vi "PostCopyScripting.vi"(10 "MetaDataObj":refnum<class "MetaDataObj.lvclass">, 11 "User Project":refnum<vi>) -> ()   [LabVIEW 2016, in "MeasurementMetaData.lvclass"]
uses:
  MeasurementMetaData.lvclass
  <resource>/dialog/NewProjectWizard/MetaDataObj/MetaDataObj.lvclass
  C:/Program Files (x86)/National Instruments/LabVIEW 2016/resource/dialog/NewProjectWizard/MetaDataObj/MetaDataObj.lvclass
  <resource>/dialog/NewProjectWizard/MetaDataObj/MetaDataObj.lvclass/MetaDataObj.ctl
  MeasurementMetaData.lvclass/MeasurementMetaData.ctl
  <vilib>/Utility/EditLVProj/Edit LVProj.lvlib
  <resource>/dialog/NewProjectWizard/Project Copying/NI_NPW_Project Copying.lvlib
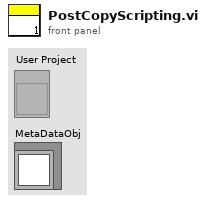
[diagram p1: front panel]
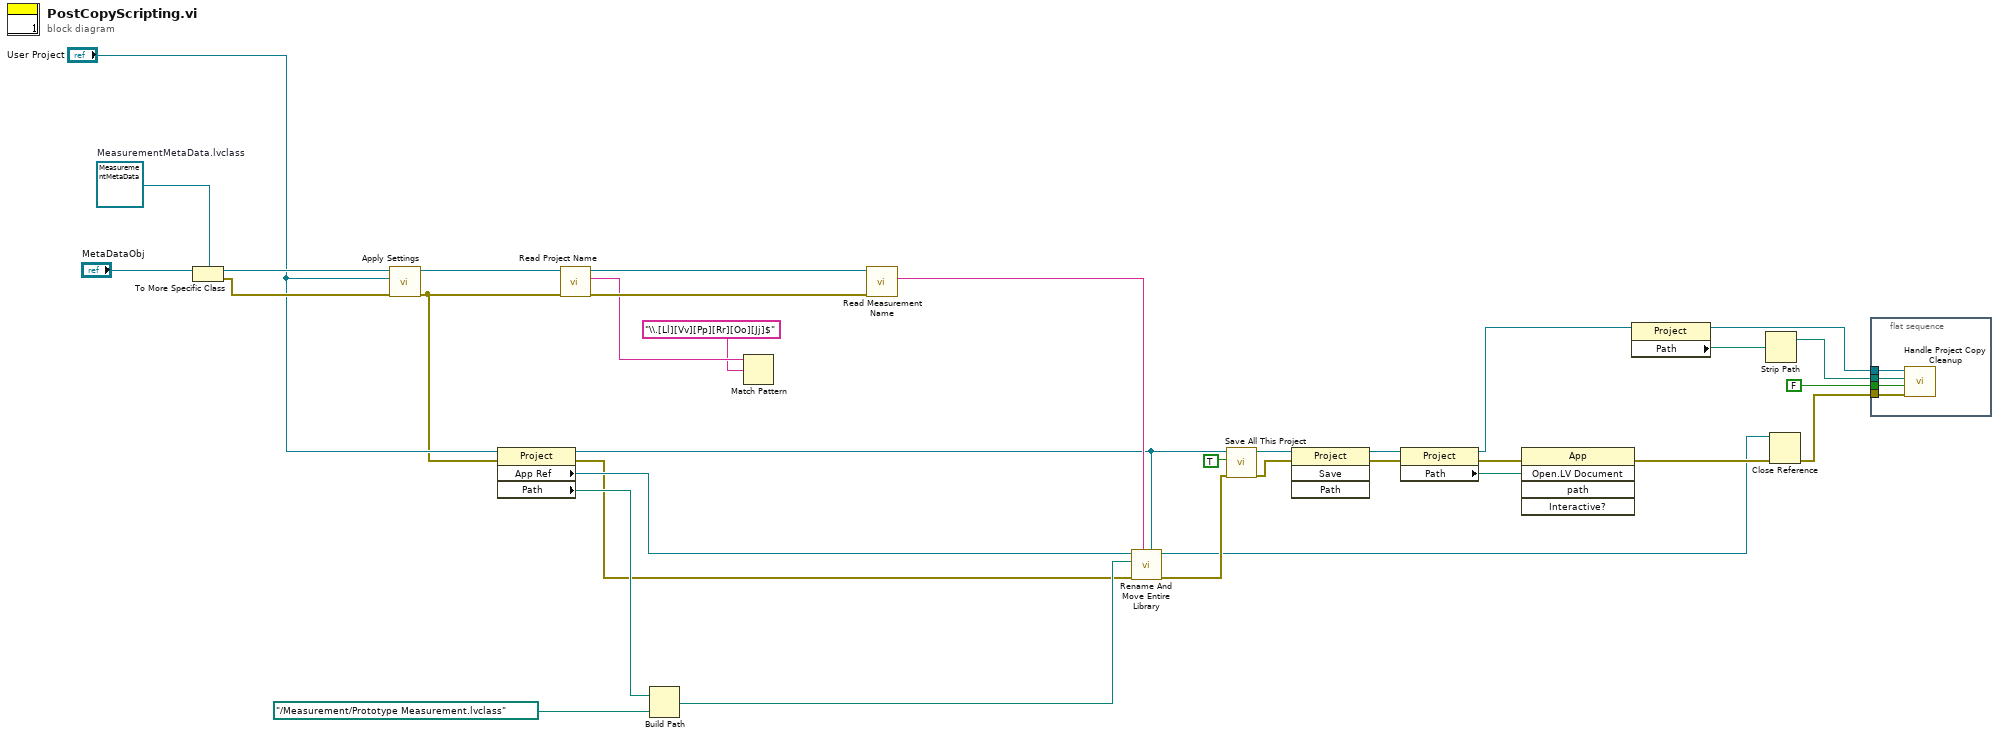
[diagram p0: block diagram]
diagram:
  w34 = refnum<class "MeasurementMetaData.lvclass"> refnum  # MeasurementMetaData.lvclass
  n1 = To More Specific Class(target class=w34, reference="MetaDataObj") -> (specific class reference=w24:refnum<class "MeasurementMetaData.lvclass">, error out=w23:errorcluster)  [unwired: 1 in]
  n2 = call "Apply Settings.vi"("error in (no error)"=w23, "User Project"="User Project", "MeasurementMetaData in"=w24) -> ("error out"=w8:errorcluster, "MeasurementMetaData out"=w10:refnum<class "MeasurementMetaData.lvclass">)  [unwired: 7 in]
  n3 = property class="Project"(reference="User Project", error in=w8) -> (reference out=w6:refnum<vi>, error out=w3:errorcluster, "App Ref"=w5:refnum<vi>, "Path"=w12:path)
  n4 = call <resource>:"Read Project Name.vi"("error in (no error)"=w8, "MetaDataObj in"=w10) -> ("error out"=w19:errorcluster, "Project Name"=w18:string, "MetaDataObj out"=w20:refnum<class "MeasurementMetaData.lvclass">)  [unwired: 7 in]
  n5 = Build Path(base path=w12, name or relative path=path "../Measurement/Prototype Measurement.lvclass" ("Path")) -> (appended path=w4:path)
  n6 = Match Pattern(string=w18, regular expression="\\.[Ll][Vv][Pp][Rr][Oo][Jj]$") -> ()  [unwired: 1 in, 4 out]
  n7 = call "Read Measurement Name.vi"("error in (no error)"=w19, "MeasurementMetaData in"=w20) -> ("Measurement Name"=w7:string)  [unwired: 7 in, 2 out]
  n8 = call "Rename And Move Entire Library.vi"("Project"=w6, "New Name Without Extension"=w7, "error in (no error)"=w3, "Library Path"=w4, "Application"=w5) -> ("error out"=w2:errorcluster, "Application out"=w1:refnum<vi>)  [unwired: 4 in, 1 out]
  n9 = call <vilib>:"Save All This Project.vi"("error in (no error)"=w2, "Exclude Dependencies? (F)"=TRUE, "Project in"=w6) -> ("error out"=w22:errorcluster, "Project out"=w31:refnum<vi>)  [unwired: 7 in]
  n10 = invoke class="Project" method="Save"(reference=w31, error in=w22) -> (reference out=w33:refnum<vi>, error out=w32:errorcluster)  [unwired: 2 in, 2 out]
  n11 = property class="Project"(reference=w33, error in=w32) -> (reference out=w14:refnum<vi>, error out=w13:errorcluster, "Path"=w16:path)
  n12 = invoke class="App" method="Open.LV Document"(error in=w13, "path"=w16) -> (error out=w15:errorcluster)  [unwired: 3 in, 4 out]
  n13 = property class="Project"(reference=w14) -> (reference out=w25:refnum<vi>, "Path"=w26:path)  [unwired: 1 in, 1 out]
  n14 = Strip Path(path=w26) -> (stripped path=w28:path)  [unwired: 1 out]
  n15 = Close Reference(reference=w1, error in (no error)=w15) -> (error out=w29:errorcluster)
  n16 = flat-sequence {
    tunnel: w29 -> [w38]
    tunnel: w28 -> [w37]
    tunnel: FALSE ("More Scripting?") -> [w36]
    tunnel: w25 -> [w35]
    frame #0 {
      n17 = call <resource>:"Handle Project Copy Cleanup.vi"("error in (no error)"=w38, "More Scripting?"=w36, "Target Path"=w37, "Project in"=w35) -> ()  [unwired: 8 in]
    }
  }
